vi "Checksum.vi"(1 "INPUT_Array":u8[](array[numeric]) format="%x") -> (0 "OUTPUT_Array":u8[](array[numeric]) format="%x")   [LabVIEW 2014]
panel:
  out "SUM":u16
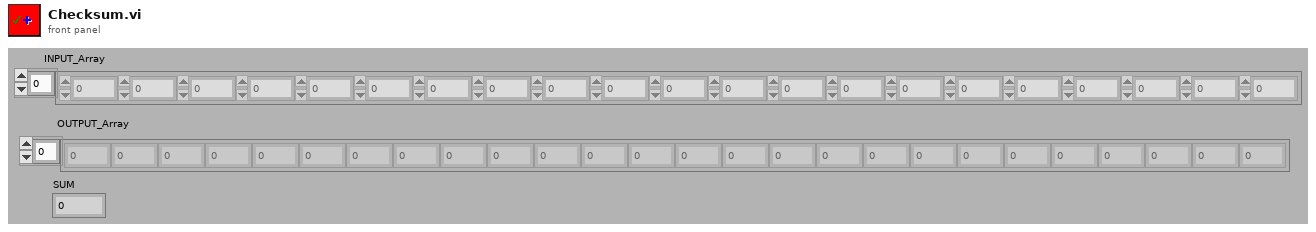
[diagram p1: front panel]
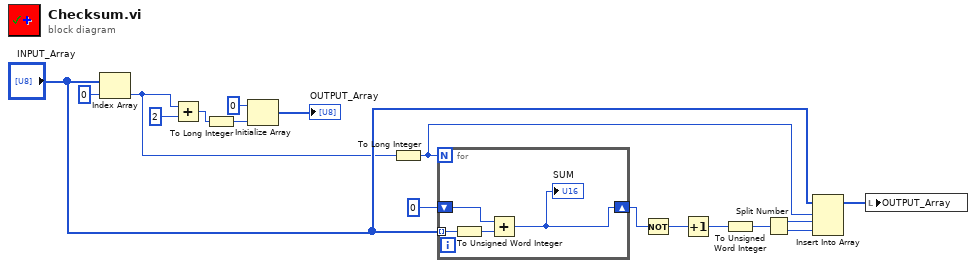
[diagram p0: block diagram]
diagram:
  n1 = Index Array(array="INPUT_Array", index=0) -> (element=w2:u8)
  n2 = Add(x=w2, y=u8 2) -> (x+y=w16:u8)
  n3 = To Long Integer(number=w16) -> (32bit integer=w17:i32)
  n4 = Initialize Array(u8 0 ("element"), w17) -> (→"OUTPUT_Array":u8[])
  n5 = To Long Integer(number=w2) -> (32bit integer=w1:i32)
  n6 = for {
    N: w1 -> [_]
    tunnel: "INPUT_Array" -> [w20] mode=indexing
    shift-right: [w18] -> w3
    shift-left: u16 0 ("Numeric") -> [w19]
    n7 = To Unsigned Word Integer(number=w20) -> (unsigned 16bit integer=w21:u16)
    n8 = Add(x=w19, y=w21) -> (x+y=w18:u16)
    "SUM" <- w18
  }
  n9 = Not(x=w3) -> (.not. x?=w10:u16)
  n10 = Increment(x=w10) -> (x+1=w9:u16)
  n11 = To Unsigned Word Integer(number=w9) -> (unsigned 16bit integer=w8:u16)
  n12 = Split Number(x=w8) -> (hi(x)=w7:u8, lo(x)=w6:u8)
  n13 = Insert Into Array(array="INPUT_Array", index=w1, new element #1=w7, new element #2=w6) -> (w11:u8[])
  n14 = local write "OUTPUT_Array"(w11) -> ()
